vi "CLOSE EXCEL.vi"(6 "SAVE":bool, 9 "File Path":path, 10 "WORKBOOK REF IN":refnum<k7>, 11 "APPLICATION REF IN":refnum<k7>) -> ()   [LabVIEW 2021]
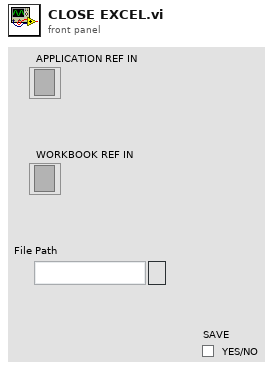
[diagram p1: front panel]
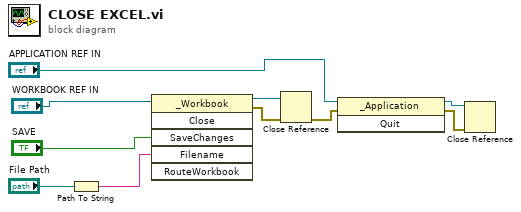
[diagram p0: block diagram]
diagram:
  n1 = Path To String(path="File Path") -> (string=w1:string)
  n2 = invoke class="_Workbook" method="Close"(reference="WORKBOOK REF IN", "SaveChanges"="SAVE", "Filename"=w1) -> (reference out=w4:refnum<k7>, error out=w5:errorcluster)  [unwired: 3 in, 4 out]
  n3 = Close Reference(reference=w4, error in (no error)=w5) -> (error out=w3:errorcluster)
  n4 = invoke class="_Application" method="Quit"(reference="APPLICATION REF IN", error in=w3) -> (reference out=w10:refnum<k7>, error out=w9:errorcluster)  [unwired: 1 in, 1 out]
  n5 = Close Reference(reference=w10, error in (no error)=w9) -> ()  [unwired: 1 out]
